vi "Goo02_F.vi"(10 "ColorSensor 2":dbl[](array[numeric]), 11 "클러스터":T1) -> ()   [LabVIEW 2014]
uses:
  <vilib>/myRIO/Instrument Drivers/Onboard IO/AI/vis/Read.vi
  <vilib>/myRIO/Instrument Drivers/Onboard IO/AI/vis/Smart Open.vi
  <vilib>/Utility/error.llb/Error Cluster From Error Code.vi
  <vilib>/myRIO/Common/Instrument Driver Framework/myRIO v1.0/AI/vis/myRIO v1.0 Read AI.vi
panel:
  in  "몇초동안 못맞추면":u32=10000
  in  "뒤이동시간":u32=500
  in  "앞":u32=100
  in  "Select Servo 6":string(combo)="Servo 6"
  in  "Select Servo 5":string(combo)="Servo 5"
  in  "Select Servo 4":string(combo)="Servo 4"
  in  "서브 컨트롤":i32=1
  in  "흰색과 흑색 차이값":dbl=0.3
  # "앞의 검은선 수평 맞추기"
  # "두 값의 차이가 이 값보다 작으면 멈춘다"
  # "第 : 4"
  # "뒤 방향 : 0"
  # "오른쪽 : 5"
  # "앞 방향 : 240"
  # "왼쪽 : 6"
  # "앞 방향: 120"
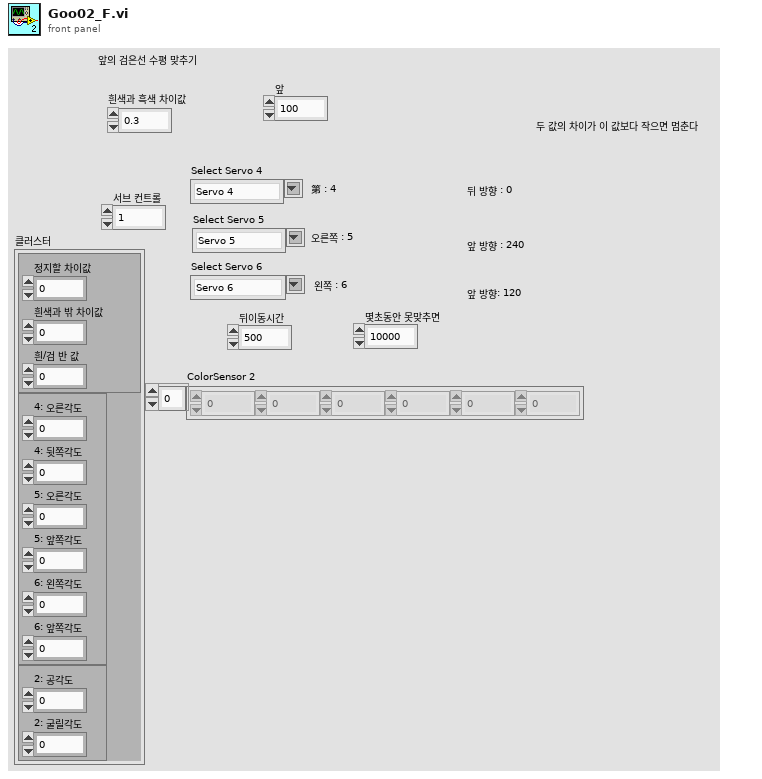
[diagram p1: front panel]
types:
  T1 = cluster{cluster{"정지할 차이값":dbl, "흰색과 밖 차이값":dbl, "흰/검 반 값 ":dbl}, cluster{"4: 오른각도":dbl, "4: 뒷쪽각도":dbl, "5: 오른각도":dbl, "5: 앞쪽각도":dbl, "6: 왼쪽각도":dbl, "6: 앞쪽각도":dbl}, cluster{"2: 공각도":dbl, "2: 굴릴각도":dbl}}
  T2 = cluster{"정지할 차이값":dbl, "흰색과 밖 차이값":dbl, "흰/검 반 값 ":dbl}
  T3 = cluster{"4: 오른각도":dbl, "4: 뒷쪽각도":dbl, "5: 오른각도":dbl, "5: 앞쪽각도":dbl, "6: 왼쪽각도":dbl, "6: 앞쪽각도":dbl}
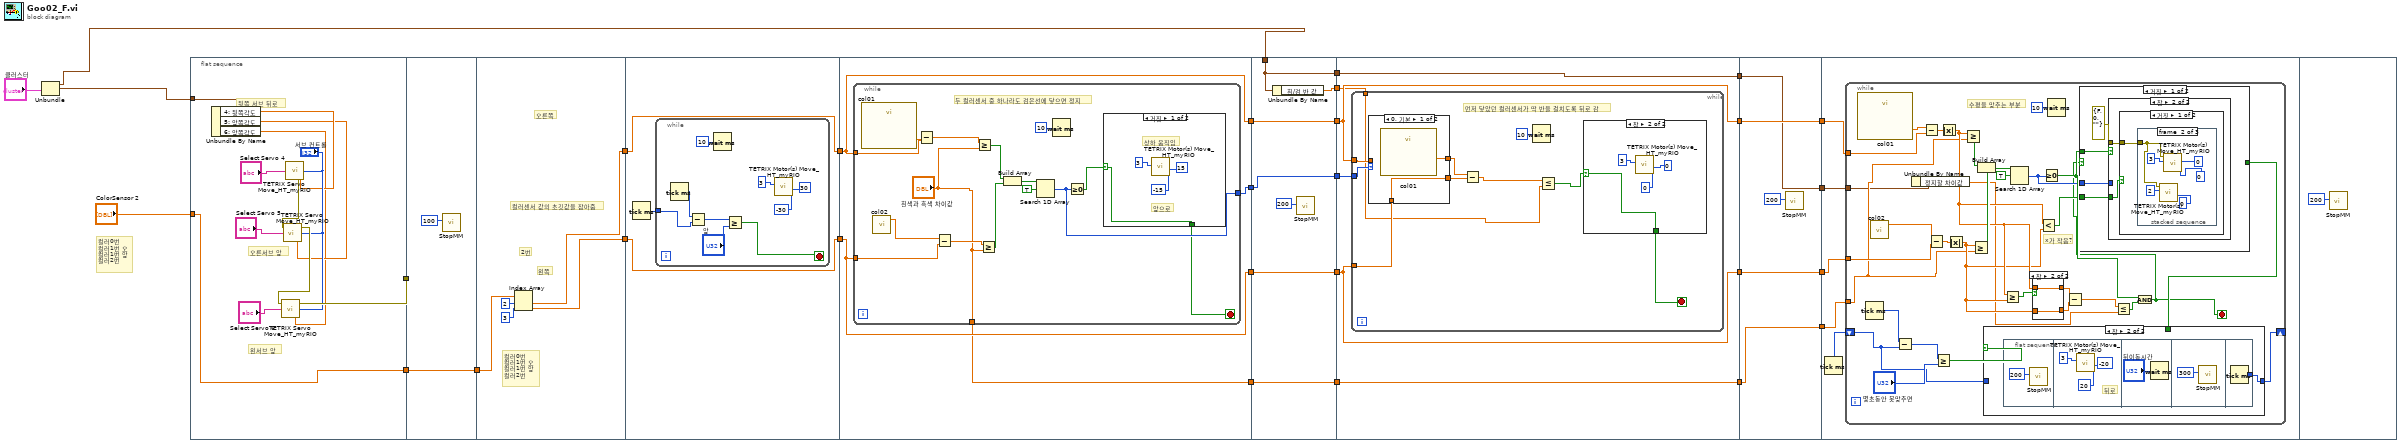
[diagram p0: block diagram]
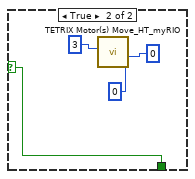
[diagram p2: hidden frame]
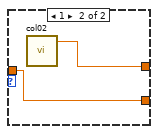
[diagram p3: hidden frame]
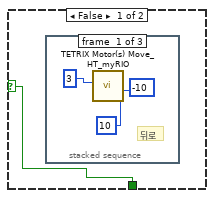
[diagram p4: hidden frame]
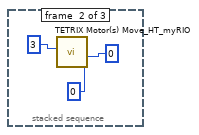
[diagram p5: hidden frame]
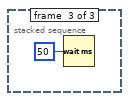
[diagram p6: hidden frame]
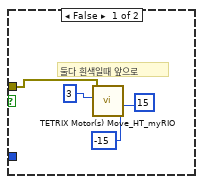
[diagram p8: hidden frame]
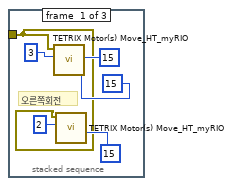
[diagram p9: hidden frame]
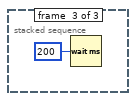
[diagram p10: hidden frame]
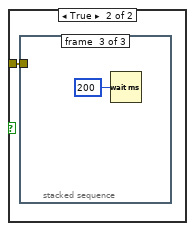
[diagram p11: hidden frame]
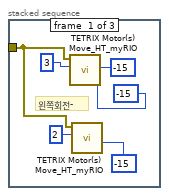
[diagram p12: hidden frame]
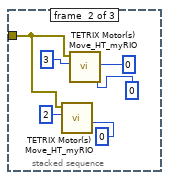
[diagram p13: hidden frame]
diagram:
  # "컬러0번\n컬러1번 오\n컬러1번 앞\n컬러2번"
  n1 = Unbundle("클러스터") -> (w7:T2, w13:T3)  [unwired: 1 out]
  n2 = flat-sequence {
    tunnel: [w36] -> w19
    tunnel: w13 -> [w34]
    tunnel: [w30] -> w2
    tunnel: "ColorSensor 2" -> [w30]
    tunnel: w19 -> [_]
    tunnel: [w42] -> w3
    tunnel: w2 -> [w42]
    tunnel: [w45] -> w18
    tunnel: [w44] -> w17
    tunnel: w3 -> [w48]
    tunnel: w18 -> [w51]
    tunnel: [w51] -> w16
    tunnel: w17 -> [w50]
    tunnel: [w50] -> w15
    tunnel: w16 -> [w63]
    tunnel: w15 -> [w64]
    tunnel: [w64] -> w29
    tunnel: [w63] -> w28
    tunnel: [w62] -> w20
    tunnel: [w61] -> w10
    tunnel: w29 -> [w94]
    tunnel: [w94] -> w27
    tunnel: w28 -> [w93]
    tunnel: [w93] -> w26
    tunnel: [w92] -> w21
    tunnel: w20 -> [w92]
    tunnel: [w89] -> w12
    tunnel: [w90] -> w11
    tunnel: w10 -> [w90]
    tunnel: w7 -> [w88]
    tunnel: [w88] -> w6
    tunnel: w27 -> [w99]
    tunnel: [w99] -> w25
    tunnel: w26 -> [w100]
    tunnel: [w100] -> w23
    tunnel: w21 -> [w98]
    tunnel: w12 -> [w97]
    tunnel: w11 -> [w96]
    tunnel: [w96] -> w8
    tunnel: w6 -> [w95]
    tunnel: [w95] -> w4
    tunnel: w25 -> [w131]
    tunnel: [w131] -> w24
    tunnel: w23 -> [w130]
    tunnel: [w130] -> w22
    tunnel: [w128] -> w9
    tunnel: w8 -> [w128]
    tunnel: [w127] -> w5
    tunnel: w4 -> [w127]
    tunnel: w24 -> [w135]
    tunnel: w22 -> [w136]
    tunnel: w9 -> [w133]
    tunnel: w5 -> [w132]
    frame #0 {
      # "오른서브 앞"
      # "뒷쪽 서브 뒤로"
      # "왼서브 앞"
      n3 = Unbundle By Name(w34) -> ("4: 뒷쪽각도"=w33:dbl, "5: 앞쪽각도"=w32:dbl, "6: 앞쪽각도"=w31:dbl)
      n4 = call <vilib>:"TETRIX Servo Move_HT_myRIO.vi"("Servo Position (0 - 255)"=w33, "Controller Daisy Chain Position (1 - 4)"="서브 컨트롤", "Select Servo"="Select Servo 4") -> ("error out"=w38:errorcluster)  [unwired: 2 in]
      n5 = call <vilib>:"TETRIX Servo Move_HT_myRIO.vi"("Servo Position (0 - 255)"=w32, "Controller Daisy Chain Position (1 - 4)"="서브 컨트롤", "Select Servo"="Select Servo 5", "error in (no error)"=w38) -> ("error out"=w37:errorcluster)  [unwired: 1 in]
      n6 = call <vilib>:"TETRIX Servo Move_HT_myRIO.vi"("Servo Position (0 - 255)"=w31, "Controller Daisy Chain Position (1 - 4)"="서브 컨트롤", "Select Servo"="Select Servo 6", "error in (no error)"=w37) -> ("error out"=w36:errorcluster)  [unwired: 1 in]
    }
    frame #1 {
      n7 = call "StopMM.vi"("대기 시간(ms)"=u32 100) -> ()  [unwired: 11 in]
    }
    frame #2 {
      # "컬러0번\n컬러1번 오\n컬러1번 앞\n컬러2번"
      # "왼쪽"
      # "오른쪽"
      # "컬러센서 값의 초깃값을 잡아줌"
      # "2번"
      n8 = Index Array(array=w48, index #1=2 ("인덱스"), index #2=3 ("인덱스")) -> (element #1=w45:dbl, element #2=w44:dbl)
    }
    frame #3 {
      n9 = Tick Count (ms)() -> (millisecond timer value=w49:u32)
      n10 = while {
        tunnel: w49 -> [w56]
        stop <- w53 stop-if-true
        n11 = Tick Count (ms)() -> (millisecond timer value=w57:u32)
        n12 = Subtract(x=w57, y=w56) -> (x-y=w55:u32)
        n13 = Wait (ms)(milliseconds to wait=u32 10 ("대기 시간(ms)")) -> ()  [unwired: 1 out]
        n14 = Greater Or Equal?(x=w55, y="앞") -> (x >= y?=w53:bool)
        n15 = call <vilib>:"TETRIX Motor(s) Move_HT_myRIO.vi"("Motor 2 Power (-100 to 100)\n0 = Stop/Brake\n-128 = Stop/Coast"=i8 -30 ("Motor 2 Power (-100 to 100)\n0 = Stop/Brake\n-128 = Stop/Coast"), "Motor 1 Power (-100 to 100)\n0 = Stop/Brake\n-128 = Stop/Coast"=i8 30 ("Motor 1 Power (-100 to 100)\n0 = Stop/Brake\n-128 = Stop/Coast"), "Controller Daisy Chain Position: 1 - 4"=u8 3) -> ()  [unwired: 6 in, 1 out]
      }
    }
    frame #4 {
      n16 = while {
        tunnel: w64 -> [w79]
        tunnel: w63 -> [w78]
        tunnel: [w68] -> w62
        tunnel: ["흰색과 흑색 차이값"] -> w61
        stop <- w65 stop-if-true
        # "두 컬러센서 중 하나라도 검은선에 닿으면 정지"
        n17 = call "col01.vi"() -> ("Col01 (B/AI1 (Pin 5))"=w70:dbl)  [unwired: 26 in, 1 out]
        n18 = call "col02.vi"() -> ("Col02 (B/AI2 (Pin 7))"=w69:dbl)  [unwired: 26 in, 1 out]
        n19 = Subtract(x=w70, y=w78) -> (x-y=w77:dbl)
        n20 = Subtract(x=w69, y=w79) -> (x-y=w76:dbl)
        n21 = Greater Or Equal?(x=w77, y="흰색과 흑색 차이값") -> (x >= y?=w75:bool)
        n22 = Greater Or Equal?(x=w76, y="흰색과 흑색 차이값") -> (x >= y?=w74:bool)
        n23 = Build Array(w75, w74) -> (w73:bool[])
        n24 = Search 1D Array(1D array=w73, element=TRUE ("원소")) -> (index of element=w68:i32)  [unwired: 1 in]
        n25 = Wait (ms)(milliseconds to wait=u32 10 ("대기 시간(ms)")) -> ()  [unwired: 1 out]
        n26 = Greater Or Equal To 0?(x=w68) -> (x >= 0?=w66:bool)
        n27 = case shown="거짓" w66 {
          selector: w66 -> [w80 w84]
          tunnel: [w80 w84] -> w65
          frame False {
            # "앞으로"
            # "상하 움직임"
            n28 = call <vilib>:"TETRIX Motor(s) Move_HT_myRIO.vi"("Motor 2 Power (-100 to 100)\n0 = Stop/Brake\n-128 = Stop/Coast"=i8 -15 ("Motor 2 Power (-100 to 100)\n0 = Stop/Brake\n-128 = Stop/Coast"), "Motor 1 Power (-100 to 100)\n0 = Stop/Brake\n-128 = Stop/Coast"=i8 15 ("Motor 1 Power (-100 to 100)\n0 = Stop/Brake\n-128 = Stop/Coast"), "Controller Daisy Chain Position: 1 - 4"=u8 3) -> ()  [unwired: 6 in, 1 out]
          }
          frame True {
            n29 = call <vilib>:"TETRIX Motor(s) Move_HT_myRIO.vi"("Motor 2 Power (-100 to 100)\n0 = Stop/Brake\n-128 = Stop/Coast"=i8 0 ("Motor 2 Power (-100 to 100)\n0 = Stop/Brake\n-128 = Stop/Coast"), "Motor 1 Power (-100 to 100)\n0 = Stop/Brake\n-128 = Stop/Coast"=i8 0 ("Motor 1 Power (-100 to 100)\n0 = Stop/Brake\n-128 = Stop/Coast"), "Controller Daisy Chain Position: 1 - 4"=u8 3) -> ()  [unwired: 6 in, 1 out]
          }
        }
      }
    }
    frame #5 {
      n30 = Unbundle By Name(w88) -> ("흰/검 반 값"=w89:dbl)
      n31 = call "StopMM.vi"("대기 시간(ms)"=u32 200) -> ()  [unwired: 11 in]
    }
    frame #6 {
      n32 = while {
        tunnel: w99 -> [w106]
        tunnel: w100 -> [w107]
        tunnel: w98 -> [w105]
        tunnel: w97 -> [w101]
        stop <- w104 stop-if-true
        # "먼저 닿았던 컬러센서가 딱 반을 걸치도록 뒤로 감"
        n33 = case shown="0, 기본" w105 {
          tunnel: [w111 w113] -> w110
          tunnel: [w112 w114] -> w108
          tunnel: w107 -> [_ w114]
          tunnel: w106 -> [w112 _]
          frame 0, Default {
            n34 = call "col01.vi"() -> ("Col01 (B/AI1 (Pin 5))"=w111:dbl)  [unwired: 26 in, 1 out]
          }
          frame 1 {
            n35 = call "col02.vi"() -> ("Col02 (B/AI2 (Pin 7))"=w113:dbl)  [unwired: 26 in, 1 out]
          }
        }
        n36 = Subtract(x=w110, y=w108) -> (x-y=w102:dbl)
        n37 = Wait (ms)(milliseconds to wait=u32 10 ("대기 시간(ms)")) -> ()  [unwired: 1 out]
        n38 = Less Or Equal?(x=w102, y=w101) -> (x <= y?=w103:bool)
        n39 = case shown="참" w103 {
          selector: w103 -> [w115 w123]
          tunnel: [w115 w123] -> w104
          frame False {
            n40 = stacked-sequence {
              frame #0 {
                # "뒤로"
                n41 = call <vilib>:"TETRIX Motor(s) Move_HT_myRIO.vi"("Motor 2 Power (-100 to 100)\n0 = Stop/Brake\n-128 = Stop/Coast"=i8 10 ("Motor 2 Power (-100 to 100)\n0 = Stop/Brake\n-128 = Stop/Coast"), "Motor 1 Power (-100 to 100)\n0 = Stop/Brake\n-128 = Stop/Coast"=i8 -10 ("Motor 1 Power (-100 to 100)\n0 = Stop/Brake\n-128 = Stop/Coast"), "Controller Daisy Chain Position: 1 - 4"=u8 3) -> ()  [unwired: 6 in, 1 out]
              }
              frame #1 {
                n42 = call <vilib>:"TETRIX Motor(s) Move_HT_myRIO.vi"("Motor 2 Power (-100 to 100)\n0 = Stop/Brake\n-128 = Stop/Coast"=i8 0 ("Motor 2 Power (-100 to 100)\n0 = Stop/Brake\n-128 = Stop/Coast"), "Motor 1 Power (-100 to 100)\n0 = Stop/Brake\n-128 = Stop/Coast"=i8 0 ("Motor 1 Power (-100 to 100)\n0 = Stop/Brake\n-128 = Stop/Coast"), "Controller Daisy Chain Position: 1 - 4"=u8 3) -> ()  [unwired: 6 in, 1 out]
              }
              frame #2 {
                n43 = Wait (ms)(milliseconds to wait=u32 50 ("대기 시간(ms)")) -> ()  [unwired: 1 out]
              }
            }
          }
          frame True {
            n44 = call <vilib>:"TETRIX Motor(s) Move_HT_myRIO.vi"("Motor 2 Power (-100 to 100)\n0 = Stop/Brake\n-128 = Stop/Coast"=i8 0 ("Motor 2 Power (-100 to 100)\n0 = Stop/Brake\n-128 = Stop/Coast"), "Motor 1 Power (-100 to 100)\n0 = Stop/Brake\n-128 = Stop/Coast"=i8 0 ("Motor 1 Power (-100 to 100)\n0 = Stop/Brake\n-128 = Stop/Coast"), "Controller Daisy Chain Position: 1 - 4"=u8 3) -> ()  [unwired: 6 in, 1 out]
          }
        }
      }
    }
    frame #7 {
      n45 = call "StopMM.vi"("대기 시간(ms)"=u32 200) -> ()  [unwired: 11 in]
    }
    frame #8 {
      n46 = Tick Count (ms)() -> (millisecond timer value=w134:u32)
      n47 = while {
        tunnel: w135 -> [w168]
        tunnel: w136 -> [w167]
        shift-right: [w141] -> _
        shift-left: w134 -> [w142]
        tunnel: w133 -> [w140]
        tunnel: w132 -> [w139]
        stop <- w137 stop-if-true
        # "x가 작음?"
        # "수평을 맞추는 부분"
        n48 = call "col01.vi"() -> ("Col01 (B/AI1 (Pin 5))"=w160:dbl)  [unwired: 26 in, 1 out]
        n49 = Tick Count (ms)() -> (millisecond timer value=w147:u32)
        n50 = call "col02.vi"() -> ("Col02 (B/AI2 (Pin 7))"=w152:dbl)  [unwired: 26 in, 1 out]
        n51 = Subtract(x=w147, y=w142) -> (x-y=w146:u32)
        n52 = Unbundle By Name(w139) -> ("정지할 차이값"=w138:dbl)
        n53 = Subtract(x=w160, y=w167) -> (x-y=w154:dbl)
        n54 = Subtract(x=w152, y=w168) -> (x-y=w153:dbl)
        n55 = Greater Or Equal?(x=w146, y="몇초동안 못맞추면") -> (x >= y?=w145:bool)
        n56 = Absolute Value(x=w154) -> (abs(x)=w150:dbl)
        n57 = Absolute Value(x=w153) -> (abs(x)=w149:dbl)
        n58 = Greater Or Equal?(x=w150, y=w140) -> (x >= y?=w166:bool)
        n59 = Greater Or Equal?(x=w149, y=w140) -> (x >= y?=w165:bool)
        n60 = Build Array(w166, w165) -> (w164:bool[])
        n61 = Greater Or Equal?(x=w150, y=w149) -> (x >= y?=w157:bool)
        n62 = Search 1D Array(1D array=w164, element=TRUE ("원소")) -> (index of element=w148:i32)  [unwired: 1 in]
        n63 = case shown="참" w157 {
          tunnel: [w217 w220] -> w156
          tunnel: w150 -> [w218 w220]
          tunnel: w149 -> [w217 w219]
          tunnel: [w218 w219] -> w155
          frame False {
          }
          frame True {
          }
        }
        n64 = Less?(x=w150, y=w149) -> (x < y?=w151:bool)
        n65 = Greater Or Equal To 0?(x=w148) -> (x >= 0?=w159:bool)
        n66 = Wait (ms)(milliseconds to wait=u32 10 ("대기 시간(ms)")) -> ()  [unwired: 1 out]
        n67 = Subtract(x=w156, y=w155) -> (x-y=w158:dbl)
        n68 = Less Or Equal?(x=w158, y=w138) -> (x <= y?=w161:bool)
        n69 = And(x=w159, y=w161) -> (x .and. y?=w137:bool)
        n70 = case shown="거짓" w137 {
          selector: w137 -> [_ w216]
          tunnel: w159 -> [w181 _]
          tunnel: w151 -> [w180 _]
          tunnel: w148 -> [w179 _]
          tunnel: [_ w216] -> w143
          frame False {
            n71 = case shown="참" w181 {
              tunnel: w180 -> [_ w186]
              tunnel: w179 -> [_ _]
              tunnel: errorcluster {"status"=FALSE, "code"=0, "source"=""} ("error in (no error)") -> [w182 w187]
              frame False {
                # "둘다 흰색일때 앞으로"
                n72 = call <vilib>:"TETRIX Motor(s) Move_HT_myRIO.vi"("Motor 2 Power (-100 to 100)\n0 = Stop/Brake\n-128 = Stop/Coast"=i8 -15 ("Motor 2 Power (-100 to 100)\n0 = Stop/Brake\n-128 = Stop/Coast"), "Motor 1 Power (-100 to 100)\n0 = Stop/Brake\n-128 = Stop/Coast"=i8 15 ("Motor 1 Power (-100 to 100)\n0 = Stop/Brake\n-128 = Stop/Coast"), "Controller Daisy Chain Position: 1 - 4"=u8 3, "error in (no error)"=w182) -> ()  [unwired: 5 in, 1 out]
              }
              frame True {
                n73 = case shown="거짓" w186 {
                  tunnel: w187 -> [w188 w202]
                  frame False {
                    n74 = stacked-sequence {
                      tunnel: w188 -> [w189 w195 _]
                      frame #0 {
                        # "오른쪽회전"
                        n75 = call <vilib>:"TETRIX Motor(s) Move_HT_myRIO.vi"("Motor 2 Power (-100 to 100)\n0 = Stop/Brake\n-128 = Stop/Coast"=i8 15 ("Motor 2 Power (-100 to 100)\n0 = Stop/Brake\n-128 = Stop/Coast"), "Motor 1 Power (-100 to 100)\n0 = Stop/Brake\n-128 = Stop/Coast"=i8 15 ("Motor 1 Power (-100 to 100)\n0 = Stop/Brake\n-128 = Stop/Coast"), "Controller Daisy Chain Position: 1 - 4"=u8 3, "error in (no error)"=w189) -> ()  [unwired: 5 in, 1 out]
                        n76 = call <vilib>:"TETRIX Motor(s) Move_HT_myRIO.vi"("Motor 1 Power (-100 to 100)\n0 = Stop/Brake\n-128 = Stop/Coast"=i8 15 ("Motor 1 Power (-100 to 100)\n0 = Stop/Brake\n-128 = Stop/Coast"), "Controller Daisy Chain Position: 1 - 4"=u8 2, "error in (no error)"=w189) -> ()  [unwired: 6 in, 1 out]
                      }
                      frame #1 {
                        n77 = call <vilib>:"TETRIX Motor(s) Move_HT_myRIO.vi"("Motor 1 Power (-100 to 100)\n0 = Stop/Brake\n-128 = Stop/Coast"=i8 0 ("Motor 1 Power (-100 to 100)\n0 = Stop/Brake\n-128 = Stop/Coast"), "Controller Daisy Chain Position: 1 - 4"=u8 2, "error in (no error)"=w195) -> ()  [unwired: 6 in, 1 out]
                        n78 = call <vilib>:"TETRIX Motor(s) Move_HT_myRIO.vi"("Motor 2 Power (-100 to 100)\n0 = Stop/Brake\n-128 = Stop/Coast"=i8 0 ("Motor 2 Power (-100 to 100)\n0 = Stop/Brake\n-128 = Stop/Coast"), "Motor 1 Power (-100 to 100)\n0 = Stop/Brake\n-128 = Stop/Coast"=i8 0 ("Motor 1 Power (-100 to 100)\n0 = Stop/Brake\n-128 = Stop/Coast"), "Controller Daisy Chain Position: 1 - 4"=u8 3, "error in (no error)"=w195) -> ()  [unwired: 5 in, 1 out]
                      }
                      frame #2 {
                        n79 = Wait (ms)(milliseconds to wait=u32 200 ("대기 시간(ms)")) -> ()  [unwired: 1 out]
                      }
                    }
                  }
                  frame True {
                    n80 = stacked-sequence {
                      tunnel: w202 -> [w203 w209 _]
                      frame #0 {
                        # "왼쪽회전-"
                        n81 = call <vilib>:"TETRIX Motor(s) Move_HT_myRIO.vi"("Motor 2 Power (-100 to 100)\n0 = Stop/Brake\n-128 = Stop/Coast"=i8 -15 ("Motor 2 Power (-100 to 100)\n0 = Stop/Brake\n-128 = Stop/Coast"), "Motor 1 Power (-100 to 100)\n0 = Stop/Brake\n-128 = Stop/Coast"=i8 -15 ("Motor 1 Power (-100 to 100)\n0 = Stop/Brake\n-128 = Stop/Coast"), "Controller Daisy Chain Position: 1 - 4"=u8 3, "error in (no error)"=w203) -> ()  [unwired: 5 in, 1 out]
                        n82 = call <vilib>:"TETRIX Motor(s) Move_HT_myRIO.vi"("Motor 1 Power (-100 to 100)\n0 = Stop/Brake\n-128 = Stop/Coast"=i8 -15 ("Motor 1 Power (-100 to 100)\n0 = Stop/Brake\n-128 = Stop/Coast"), "Controller Daisy Chain Position: 1 - 4"=u8 2, "error in (no error)"=w203) -> ()  [unwired: 6 in, 1 out]
                      }
                      frame #1 {
                        n83 = call <vilib>:"TETRIX Motor(s) Move_HT_myRIO.vi"("Motor 1 Power (-100 to 100)\n0 = Stop/Brake\n-128 = Stop/Coast"=i8 0 ("Motor 1 Power (-100 to 100)\n0 = Stop/Brake\n-128 = Stop/Coast"), "Controller Daisy Chain Position: 1 - 4"=u8 2, "error in (no error)"=w209) -> ()  [unwired: 6 in, 1 out]
                        n84 = call <vilib>:"TETRIX Motor(s) Move_HT_myRIO.vi"("Motor 2 Power (-100 to 100)\n0 = Stop/Brake\n-128 = Stop/Coast"=i8 0 ("Motor 2 Power (-100 to 100)\n0 = Stop/Brake\n-128 = Stop/Coast"), "Motor 1 Power (-100 to 100)\n0 = Stop/Brake\n-128 = Stop/Coast"=i8 0 ("Motor 1 Power (-100 to 100)\n0 = Stop/Brake\n-128 = Stop/Coast"), "Controller Daisy Chain Position: 1 - 4"=u8 3, "error in (no error)"=w209) -> ()  [unwired: 5 in, 1 out]
                      }
                      frame #2 {
                        n85 = Wait (ms)(milliseconds to wait=u32 200 ("대기 시간(ms)")) -> ()  [unwired: 1 out]
                      }
                    }
                  }
                }
              }
            }
          }
          frame True {
          }
        }
        n86 = case shown="참" w145 {
          tunnel: w143 -> [_ _]
          tunnel: w142 -> [w169 _]
          tunnel: [w169 w170] -> w141
          frame False {
          }
          frame True {
            n87 = flat-sequence {
              tunnel: [w177] -> w170
              frame #0 {
                n88 = call "StopMM.vi"("대기 시간(ms)"=u32 200) -> ()  [unwired: 11 in]
              }
              frame #1 {
                # "뒤로"
                n89 = call <vilib>:"TETRIX Motor(s) Move_HT_myRIO.vi"("Motor 2 Power (-100 to 100)\n0 = Stop/Brake\n-128 = Stop/Coast"=i8 20 ("Motor 2 Power (-100 to 100)\n0 = Stop/Brake\n-128 = Stop/Coast"), "Motor 1 Power (-100 to 100)\n0 = Stop/Brake\n-128 = Stop/Coast"=i8 -20 ("Motor 1 Power (-100 to 100)\n0 = Stop/Brake\n-128 = Stop/Coast"), "Controller Daisy Chain Position: 1 - 4"=u8 3) -> ()  [unwired: 6 in, 1 out]
              }
              frame #2 {
                n90 = Wait (ms)(milliseconds to wait="뒤이동시간") -> ()  [unwired: 1 out]
              }
              frame #3 {
                n91 = call "StopMM.vi"("대기 시간(ms)"=u32 300) -> ()  [unwired: 11 in]
              }
              frame #4 {
                n92 = Tick Count (ms)() -> (millisecond timer value=w177:u32)
              }
            }
          }
        }
      }
    }
    frame #9 {
      n93 = call "StopMM.vi"("대기 시간(ms)"=u32 200) -> ()  [unwired: 11 in]
    }
  }
